vi "toFloatImage.vi"(2 "value_in":u8[](array[numeric]), 3 "dim_y":i32, 4 "dim_x":i32) -> (0 "setpoint":sgl[][](array[numeric]), 1 "value_out":sgl[][](array[numeric]))   [LabVIEW 2014, in "tango.lvlib"]
uses:
  tango.lvlib
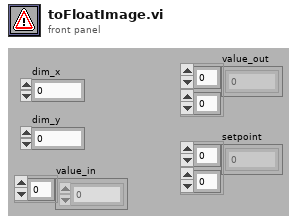
[diagram p1: front panel]
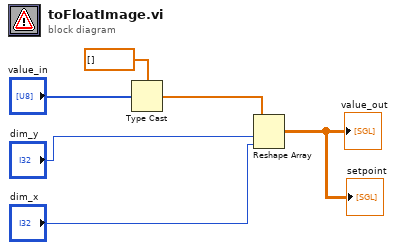
[diagram p0: block diagram]
diagram:
  n1 = Type Cast(type=sgl[] [], x="value_in") -> (*(type *) &x=w2:sgl[])
  n2 = Reshape Array(w2, "dim_y", "dim_x") -> (→"value_out" →"setpoint":sgl[][])
